vi "Dec To ASCII.vi"(11 "10进制数":dbl) -> (2 "转换后的数据（ASCII）":string)   [LabVIEW 2017]
panel:
  out "高位":string
  out "低位":string
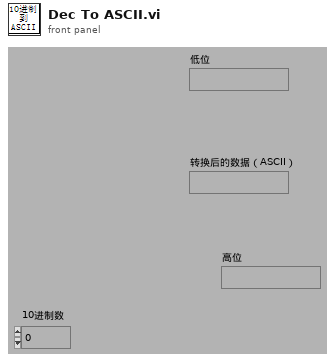
[diagram p1: front panel]
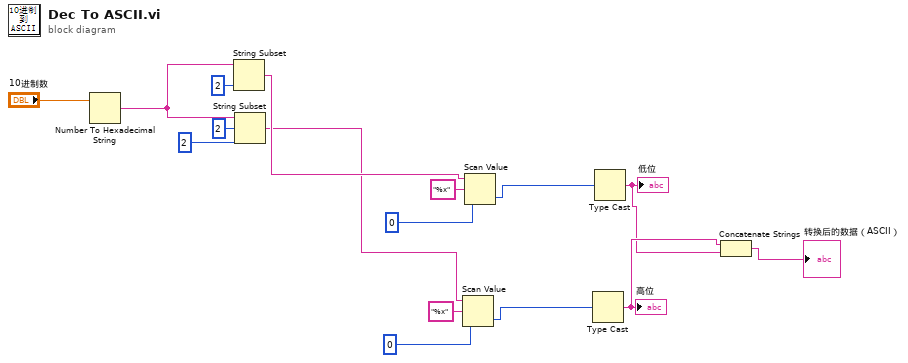
[diagram p0: block diagram]
diagram:
  n1 = Number To Hexadecimal String(2:"10进制数") -> (0:w15:string)  [unwired: 1 in]
  n2 = String Subset(string=w15, length (rest)=2 ("长度（剩余）")) -> (substring=w8:string)  [unwired: 1 in]
  n3 = String Subset(string=w15, offset (0)=2 ("偏移量(0)"), length (rest)=2 ("长度（剩余）")) -> (substring=w4:string)
  n4 = Scan Value(string=w4, format string="%x" ("格式字符串"), default (0 dbl)=u8 0 ("默认(0 dbl)")) -> (value=w7:u8)  [unwired: 1 out]
  n5 = Scan Value(string=w8, format string="%x" ("格式字符串"), default (0 dbl)=u8 0 ("默认(0 dbl)")) -> (value=w9:u8)  [unwired: 1 out]
  n6 = Type Cast(x=w7) -> (*(type *) &x=w2:string)  [unwired: 1 in]
  "高位" <- w2
  n7 = Type Cast(x=w9) -> (*(type *) &x=w1:string)  [unwired: 1 in]
  "低位" <- w1
  n8 = Concatenate Strings(w2, w1) -> (→"转换后的数据（ASCII）":string)
